vi "NaI_Readout_tdms.vi"() -> ()   [LabVIEW 2016]
doc: "Example: Configured Acquisition Auto TRIG\n\nRecommended Input Signal: 100 kHz, 4 Vpp, sine wave\n\nDevices Supported: NI 5102, NI 5911, NI 5112, NI 5620 \n(NI 5620 requires configuring 50 ohm input impedance and a 2 V vertical range)\n\nDescription:\n\nThis example is the same as the configured acquisition example included with the shipping examples, except this VI will use an immediate trigger if a timeout error is returned because no trigger is present. If a timeout occurs the code aborts and resets the session, while setting the trigger source to immediate. This example allows you use any of the available trigger sources, rather than just edge trigger as in the AutoSetup VI."
uses:
  <instrlib>/niScope/Acquire/Fetch/niScope Multi Fetch.vi
panel:
  out "Histogram":dynamicdata(graph)
  in  "resource name":refnum<k15>="PXI1Slot8"
  in  "Operator":string="Hsin-Yeh"
  in  "Target Total Events":i32=10000
  in  "file path":path=path "C:/Users/NTU/Desktop/Chih-Ping/NaI0827/1-haveNumber/Co60/Co60_5.tdms"
  out "Waveform from Digitizer vs. Sample Number":dbl[][](graph)=[[-0.007034295140918245, -0.005815471424873819, -0.004596647708829393, -0.0033778239927849674, -0.0033778239927849674, -0.004596647708829393, -0.007034295140918245, -0.0033778239927849674, -0.005815471424873819, -0.0033778239927849674, -0.0021590002767405414, -0.005815471424873819, -0.005815471424873819, -0.004596647708829393, -0.005815471424873819, -0.004596647708829393, -0.007034295140918245, -0.0021590002767405414, -0.005815471424873819, -0.005815471424873819, -0.0033778239927849674, -0.004596647708829393, -0.004596647708829393, -0.004596647708829393, -0.0033778239927849674, -0.0021590002767405414, -0.007034295140918245, -0.004596647708829393, -0.0033778239927849674, -0.004596647708829393, -0.0021590002767405414, -0.007034295140918245, -0.004596647708829393, -0.005815471424873819, -0.0033778239927849674, -0.0033778239927849674, -0.004596647708829393, -0.004596647708829393, -0.005815471424873819, -0.004596647708829393, -0.008253118856962671, -0.004596647708829393, -0.004596647708829393, -0.004596647708829393, -0.004596647708829393, -0.007034295140918245, -0.007034295140918245, -0.005815471424873819, -0.007034295140918245, -0.004596647708829393, -0.005815471424873819, -0.004596647708829393, -0.004596647708829393, -0.0021590002767405414, -0.007034295140918245, 0.0002786471553483105, -0.005815471424873819, -0.005815471424873819, -0.0033778239927849674, -0.005815471424873819, -0.004596647708829393, -0.004596647708829393, -0.005815471424873819, -0.005815471424873819, -0.005815471424873819, -0.005815471424873819, -0.0033778239927849674, -0.007034295140918245, -0.004596647708829393, -0.004596647708829393, -0.004596647708829393, -0.0033778239927849674, -0.005815471424873819, -0.0033778239927849674, -0.004596647708829393, -0.005815471424873819, -0.005815471424873819, -0.0021590002767405414, -0.004596647708829393, -0.004596647708829393, -0.004596647708829393, -0.0033778239927849674, -0.009471942573007097, -0.004596647708829393, -0.007034295140918245, -0.004596647708829393, -0.007034295140918245, -0.0033778239927849674, -0.0033778239927849674, -0.004596647708829393, -0.005815471424873819, -0.0021590002767405414, -0.005815471424873819, -0.005815471424873819, -0.004596647708829393, -0.004596647708829393, -0.007034295140918245, -0.0033778239927849674, -0.005815471424873819, -0.008253118856962671, -0.007034295140918245, -0.004596647708829393, -0.0033778239927849674, -0.004596647708829393, -0.008253118856962671, -0.0033778239927849674, -0.007034295140918245, -0.0033778239927849674, -0.0033778239927849674, -0.004596647708829393, -0.007034295140918245, -0.004596647708829393, -0.0033778239927849674, -0.007034295140918245, -0.004596647708829393, -0.004596647708829393, -0.007034295140918245, -0.004596647708829393, -0.005815471424873819, -0.004596647708829393, -0.007034295140918245, -0.004596647708829393, -0.004596647708829393, -0.0033778239927849674, -0.005815471424873819, -0.007034295140918245, -0.005815471424873819, -0.005815471424873819, -0.004596647708829393, -0.005815471424873819, -0.004596647708829393, -0.0033778239927849674, -0.0033778239927849674, -0.005815471424873819, -0.005815471424873819, -0.004596647708829393, -0.004596647708829393, -0.005815471424873819, -0.004596647708829393, -0.005815471424873819, -0.005815471424873819, -0.0021590002767405414, -0.0033778239927849674, -0.004596647708829393, -0.007034295140918245, -0.005815471424873819, -0.005815471424873819, -0.004596647708829393, -0.007034295140918245, -0.005815471424873819, -0.0033778239927849674, -0.0009401765606961154, -0.004596647708829393, -0.004596647708829393, -0.0033778239927849674, -0.0021590002767405414, -0.005815471424873819, -0.004596647708829393, -0.005815471424873819, 0.008810413167659292, 0.06000100924152518, 0.07584571755010272, 0.08559630727845813, 0.08803395471054698, 0.09169042585868026, 0.08803395471054698, 0.0892527784265914, 0.08803395471054698, 0.09169042585868026, 0.09290924957472468, 0.0892527784265914, 0.08803395471054698, 0.09047160214263583, 0.0892527784265914, 0.09169042585868026, 0.08681513099450255, 0.0892527784265914, 0.08803395471054698, 0.08559630727845813, 0.08681513099450255, 0.0892527784265914, 0.08803395471054698, 0.08315865984636928, 0.08559630727845813, 0.08559630727845813, 0.08559630727845813, 0.08315865984636928, 0.08559630727845813, 0.0843774835624137, 0.08315865984636928, 0.08193983613032485, 0.08315865984636928, 0.0843774835624137, 0.079502188698236, 0.08315865984636928, 0.079502188698236, 0.0843774835624137, 0.0843774835624137, 0.079502188698236, 0.07828336498219157, 0.08072101241428042, 0.079502188698236, 0.07828336498219157, 0.079502188698236, 0.07706454126614715, 0.07706454126614715, 0.079502188698236, 0.079502188698236, 0.07828336498219157, 0.0746268938340583, 0.07828336498219157, 0.07584571755010272, 0.07218924640196944, 0.079502188698236, 0.07340807011801387, 0.07584571755010272, 0.0746268938340583, 0.07340807011801387, 0.07218924640196944, 0.07340807011801387, 0.07218924640196944, 0.07340807011801387, 0.07097042268592502, 0.07097042268592502, 0.0746268938340583, 0.07218924640196944, 0.07097042268592502, 0.07340807011801387, 0.06975159896988059, 0.06853277525383616, 0.07340807011801387, 0.06731395153779174, 0.07097042268592502, 0.06975159896988059, 0.07097042268592502, 0.06853277525383616, 0.06853277525383616, 0.06731395153779174, 0.06731395153779174, 0.06609512782174731, 0.06609512782174731, 0.06609512782174731, 0.06975159896988059, 0.06487630410570289, 0.06487630410570289, 0.06731395153779174, 0.06609512782174731, 0.06487630410570289, 0.062438656673614035, 0.06365748038965846, 0.06731395153779174, 0.06731395153779174, 0.062438656673614035, 0.06000100924152518, 0.06121983295756961, 0.06121983295756961, 0.06365748038965846, 0.06365748038965846, 0.062438656673614035, 0.06000100924152518, 0.062438656673614035, 0.06121983295756961, 0.05878218552548076, 0.05878218552548076, 0.06121983295756961, 0.05878218552548076, 0.06121983295756961, 0.06000100924152518, 0.06000100924152518, 0.05756336180943633, 0.05878218552548076, 0.05878218552548076, 0.056344538093391905, 0.056344538093391905, 0.05756336180943633, 0.06000100924152518, 0.05756336180943633, 0.05878218552548076, 0.06000100924152518, 0.056344538093391905, 0.056344538093391905, 0.05512571437734748, 0.05512571437734748, 0.05512571437734748, 0.05512571437734748, 0.05512571437734748, 0.05268806694525863, 0.05390689066130305, 0.05268806694525863, 0.05512571437734748, 0.0514692432292142, 0.05390689066130305, 0.0514692432292142, 0.05268806694525863, 0.05268806694525863, 0.05268806694525863, 0.0514692432292142, 0.050250419513169775, 0.04903159579712535, 0.04903159579712535, 0.04903159579712535, 0.050250419513169775, 0.05268806694525863, 0.050250419513169775, 0.050250419513169775, 0.050250419513169775, 0.0514692432292142, 0.044156300932947645, 0.0514692432292142, 0.0465939483650365, 0.0514692432292142, 0.0465939483650365, 0.04903159579712535, 0.050250419513169775, 0.044156300932947645, 0.04903159579712535, 0.04781277208108092, 0.04781277208108092, 0.04903159579712535, 0.0465939483650365, 0.04171865350085879, 0.0465939483650365, 0.04537512464899207, 0.0465939483650365, 0.044156300932947645, 0.04781277208108092, 0.04537512464899207, 0.044156300932947645, 0.044156300932947645, 0.04781277208108092, 0.04171865350085879, 0.04171865350085879, 0.04293747721690322, 0.04293747721690322, 0.04171865350085879, 0.044156300932947645, 0.04293747721690322, 0.04171865350085879, 0.038062182352725515, 0.04537512464899207, 0.04293747721690322, 0.04049982978481437, 0.04293747721690322, 0.03928100606876994, 0.04293747721690322, 0.04049982978481437, 0.04171865350085879, 0.03928100606876994, 0.04049982978481437, 0.04049982978481437, 0.04049982978481437, 0.04171865350085879, 0.04049982978481437, 0.03928100606876994, 0.03928100606876994, 0.03928100606876994, 0.04171865350085879, 0.04049982978481437, 0.038062182352725515, 0.03684335863668109, 0.03684335863668109, 0.03928100606876994, 0.038062182352725515, 0.035624534920636663, 0.038062182352725515, 0.03928100606876994, 0.038062182352725515, 0.03684335863668109, 0.03318688748854781, 0.03928100606876994, 0.03684335863668109, 0.03318688748854781, 0.035624534920636663, 0.035624534920636663, 0.03684335863668109, 0.03440571120459224, 0.03684335863668109, 0.035624534920636663, 0.03440571120459224, 0.03440571120459224, 0.03684335863668109, 0.03318688748854781, 0.035624534920636663, 0.03318688748854781, 0.038062182352725515, 0.035624534920636663, 0.035624534920636663, 0.03440571120459224, 0.03318688748854781, 0.03440571120459224, 0.03440571120459224, 0.03318688748854781, 0.03318688748854781, 0.03318688748854781, 0.03318688748854781, 0.03318688748854781, 0.03074924005645896, 0.03074924005645896, 0.029530416340414534, 0.029530416340414534, 0.03318688748854781, 0.031968063772503386, 0.028311592624370108, 0.031968063772503386, 0.029530416340414534, 0.03074924005645896, 0.027092768908325682, 0.03074924005645896, 0.03074924005645896, 0.031968063772503386, 0.031968063772503386, 0.027092768908325682, 0.029530416340414534, 0.03074924005645896, 0.02465512147623683, 0.028311592624370108, 0.029530416340414534, 0.029530416340414534, 0.029530416340414534, 0.03074924005645896, 0.027092768908325682, 0.028311592624370108, 0.027092768908325682, 0.029530416340414534, 0.027092768908325682, 0.02465512147623683, 0.031968063772503386, 0.027092768908325682, 0.027092768908325682, 0.027092768908325682, 0.02465512147623683, 0.028311592624370108, 0.02465512147623683, 0.025873945192281256, 0.025873945192281256, 0.023436297760192404, 0.027092768908325682, 0.023436297760192404, 0.025873945192281256, 0.025873945192281256, 0.02465512147623683, 0.028311592624370108, 0.027092768908325682, 0.027092768908325682, 0.023436297760192404, 0.022217474044147978, 0.025873945192281256, 0.02465512147623683, 0.023436297760192404, 0.027092768908325682, 0.023436297760192404, 0.023436297760192404, 0.022217474044147978, 0.027092768908325682, 0.02465512147623683, 0.02465512147623683, 0.02465512147623683, 0.023436297760192404, 0.02465512147623683, 0.02465512147623683, 0.02465512147623683, 0.022217474044147978, 0.02465512147623683, 0.02465512147623683, 0.02465512147623683, 0.02465512147623683, 0.022217474044147978, 0.022217474044147978, 0.020998650328103552, 0.017342179179970274, 0.020998650328103552, 0.019779826612059126, 0.020998650328103552, 0.0185610028960147, 0.022217474044147978, 0.020998650328103552, 0.023436297760192404, 0.019779826612059126, 0.019779826612059126, 0.022217474044147978, 0.017342179179970274, 0.0185610028960147, 0.0185610028960147, 0.019779826612059126, 0.014904531747881422, 0.019779826612059126, 0.02465512147623683, 0.019779826612059126, 0.019779826612059126, 0.020998650328103552, 0.019779826612059126, 0.016123355463925848, 0.019779826612059126, 0.020998650328103552, 0.017342179179970274, 0.0185610028960147, 0.0185610028960147, 0.017342179179970274, 0.0185610028960147, 0.020998650328103552, 0.0185610028960147, 0.019779826612059126, 0.017342179179970274, 0.014904531747881422, 0.016123355463925848, 0.017342179179970274, 0.0185610028960147, 0.016123355463925848, 0.017342179179970274, 0.017342179179970274, 0.017342179179970274, 0.0185610028960147, 0.019779826612059126, 0.014904531747881422, 0.019779826612059126, 0.013685708031836996, 0.016123355463925848, 0.017342179179970274, 0.014904531747881422, 0.017342179179970274, 0.016123355463925848, 0.017342179179970274, 0.014904531747881422, 0.014904531747881422, 0.013685708031836996, 0.017342179179970274, 0.016123355463925848, 0.013685708031836996, 0.017342179179970274, 0.0185610028960147, 0.014904531747881422, 0.016123355463925848, 0.013685708031836996, 0.017342179179970274, 0.01246688431579257, 0.014904531747881422, 0.014904531747881422, 0.014904531747881422, 0.014904531747881422, 0.014904531747881422, 0.013685708031836996, 0.013685708031836996, 0.016123355463925848, 0.01246688431579257, 0.013685708031836996, 0.013685708031836996, 0.013685708031836996, 0.013685708031836996, 0.014904531747881422, 0.014904531747881422, 0.01246688431579257, 0.01246688431579257, 0.013685708031836996, 0.014904531747881422, 0.013685708031836996, 0.013685708031836996, 0.013685708031836996, 0.01246688431579257, 0.017342179179970274, 0.016123355463925848, 0.013685708031836996, 0.016123355463925848, 0.01246688431579257, 0.013685708031836996, 0.014904531747881422, 0.01246688431579257, 0.010029236883703718, 0.013685708031836996, 0.010029236883703718, 0.010029236883703718, 0.014904531747881422, 0.013685708031836996, 0.014904531747881422, 0.011248060599748144, 0.008810413167659292, 0.011248060599748144, 0.01246688431579257, 0.013685708031836996, 0.008810413167659292, 0.013685708031836996, 0.01246688431579257, 0.01246688431579257, 0.01246688431579257, 0.01246688431579257, 0.008810413167659292, 0.013685708031836996, 0.013685708031836996, 0.010029236883703718, 0.008810413167659292, 0.011248060599748144, 0.01246688431579257, 0.01246688431579257, 0.008810413167659292, 0.01246688431579257, 0.010029236883703718, 0.013685708031836996, 0.00637276573557044, 0.007591589451614866, 0.010029236883703718, 0.010029236883703718, 0.010029236883703718, 0.008810413167659292, 0.01246688431579257, 0.011248060599748144, 0.010029236883703718, 0.008810413167659292, 0.008810413167659292, 0.011248060599748144, 0.007591589451614866, 0.010029236883703718, 0.008810413167659292, 0.00637276573557044, 0.008810413167659292, 0.01246688431579257, 0.008810413167659292, 0.01246688431579257, 0.011248060599748144, 0.008810413167659292, 0.008810413167659292, 0.007591589451614866, 0.008810413167659292, 0.00637276573557044, 0.010029236883703718, 0.010029236883703718, 0.005153942019526014, 0.00637276573557044, 0.007591589451614866, 0.007591589451614866, 0.008810413167659292, 0.008810413167659292, 0.010029236883703718, 0.008810413167659292, 0.008810413167659292, 0.007591589451614866, 0.007591589451614866, 0.007591589451614866, 0.00637276573557044, 0.00637276573557044, 0.010029236883703718, 0.00637276573557044, 0.007591589451614866, 0.007591589451614866, 0.010029236883703718, 0.010029236883703718, 0.011248060599748144, 0.008810413167659292, 0.005153942019526014, 0.007591589451614866, 0.00637276573557044, 0.00637276573557044, 0.00637276573557044, 0.005153942019526014, 0.007591589451614866, 0.007591589451614866, 0.007591589451614866, 0.007591589451614866, 0.01246688431579257, 0.00637276573557044, 0.007591589451614866, 0.008810413167659292, 0.005153942019526014, 0.005153942019526014, 0.008810413167659292, 0.00637276573557044, 0.00637276573557044, 0.00637276573557044, 0.005153942019526014, 0.003935118303481588, 0.005153942019526014, 0.007591589451614866, 0.0014974708713927365, 0.005153942019526014, 0.005153942019526014, 0.005153942019526014, 0.007591589451614866, 0.003935118303481588, 0.005153942019526014, 0.003935118303481588, 0.008810413167659292, 0.003935118303481588, 0.003935118303481588, 0.003935118303481588, 0.00637276573557044, 0.005153942019526014, 0.005153942019526014, 0.005153942019526014, 0.005153942019526014, 0.007591589451614866, 0.00637276573557044, 0.00637276573557044, 0.005153942019526014, 0.00637276573557044, 0.00637276573557044, 0.00637276573557044, 0.003935118303481588, 0.003935118303481588, 0.005153942019526014, 0.005153942019526014, 0.005153942019526014, 0.008810413167659292, 0.0027162945874371625, 0.005153942019526014, 0.005153942019526014, 0.0027162945874371625, 0.003935118303481588, 0.005153942019526014, 0.003935118303481588, 0.0014974708713927365, 0.003935118303481588, 0.00637276573557044, 0.005153942019526014, 0.00637276573557044, 0.0027162945874371625, 0.003935118303481588, 0.0027162945874371625, 0.003935118303481588, 0.003935118303481588, 0.0027162945874371625, 0.007591589451614866, 0.005153942019526014, 0.003935118303481588, 0.003935118303481588, 0.005153942019526014, 0.003935118303481588, 0.0027162945874371625, 0.005153942019526014, 0.0027162945874371625, 0.00637276573557044, -0.0009401765606961154, 0.003935118303481588, 0.005153942019526014, 0.005153942019526014, 0.003935118303481588, 0.005153942019526014, 0.0002786471553483105, 0.0002786471553483105, 0.003935118303481588, 0.0014974708713927365, 0.0027162945874371625, 0.0027162945874371625, 0.0014974708713927365, 0.0027162945874371625, 0.0027162945874371625, 0.0014974708713927365, 0.0014974708713927365, 0.003935118303481588, 0.0027162945874371625, 0.0014974708713927365, 0.0027162945874371625, 0.0027162945874371625, 0.0027162945874371625, 0.005153942019526014, 0.0027162945874371625, 0.0014974708713927365, 0.003935118303481588, -0.0021590002767405414, 0.0002786471553483105, 0.005153942019526014, 0.0002786471553483105, 0.0027162945874371625, 0.0027162945874371625, 0.003935118303481588, 0.0027162945874371625, 0.0014974708713927365, -0.0009401765606961154, 0.0002786471553483105, 0.003935118303481588, 0.0002786471553483105, 0.0014974708713927365, 0.005153942019526014, 0.0027162945874371625, 0.0027162945874371625, 0.0027162945874371625, 0.003935118303481588, 0.003935118303481588, 0.0002786471553483105, 0.0027162945874371625, 0.0002786471553483105, 0.0014974708713927365, -0.0021590002767405414, 0.003935118303481588, 0.0027162945874371625, 0.0014974708713927365, 0.0027162945874371625, 0.0002786471553483105, 0.0014974708713927365, 0.0014974708713927365, 0.0002786471553483105, 0.0014974708713927365, 0.0014974708713927365, -0.0009401765606961154, 0.0014974708713927365, 0.0002786471553483105, 0.0014974708713927365, 0.0002786471553483105, 0.0002786471553483105, 0.0014974708713927365, 0.0014974708713927365, 0.0002786471553483105, -0.0009401765606961154]]
  out "Event rate (Hz)":dbl=73.3159330185636
  in  "reference position":dbl=20.0 caption="Ref Position" format="%.1f"
  out "Event Number":dbl=10000.0
  in  "Don't Write Data":bool
  in  "trigger coupling":i32(slide)=1 caption="Trigger Coupling"
  in  "trigger level":dbl=0.03 caption="Trigger Level" format="%.2f"
  in  "trigger holdoff":dbl caption="Trigger Holdoff" format="%^.4e"
  in  "trigger delay":dbl caption="Trigger Delay" format="%^.4e"
  in  "trigger slope":i32(ring) caption="Trigger Slope" items=["Positive", "Negative"]
  in  "trigger source":string(combo)="0" caption="Trigger Source"
  in  "maximum input frequency":dbl=1000000000.0 caption="Max. Input Frequency" format="%.2f"
  in  "input impedance":u32(ring)=2 caption="Input Impedance" items=["1 mega ohm", "75 ohms", "50 ohms"]
  in  "vertical coupling":u32(slide)=1 caption="Vertical\nCcoupling"
  in  "probe attenuation":dbl=1.0 caption="Probe Attenuation" format="%.1f"
  in  "vertical offset":dbl=0.5 caption="Vertical Offset" format="%.4f"
  in  "trigger type":enum16{"Edge"}(ring) caption="Trigger Type"
  out "actual sample rate":dbl=5000000.0 caption="Actual Sample Rate" format="%^.2e"
  out "actual record length":i32=800 caption="Actual Record Length"
  in  "?":bool
  in  "min record length":i32=800 caption="Min. Record Length"
  in  "min sample rate":dbl=5000000.0 caption="Min. Sample Rate" step=1000000.0 format="%^.2e"
  in  "vertical range":dbl=1.0 caption="Vertical Range (V)" format="%.2f"
  in  "channel name":string="0" caption="Channel Name(s)"
  # "Vertical"
  # "Channel"
  # "Trigger"
  # "Trigger Selection"
  # "Specific Parameters - Not all parameters \napply to all trigger types."
  # "Horizontal"
  # "Common Parameters"
  # "NI PXIe 5162 Spec : 1.5 GHz, 5 GS/s, 10-Bit\nhttps://www.ni.com/pdf/manuals/373858j.pdf"
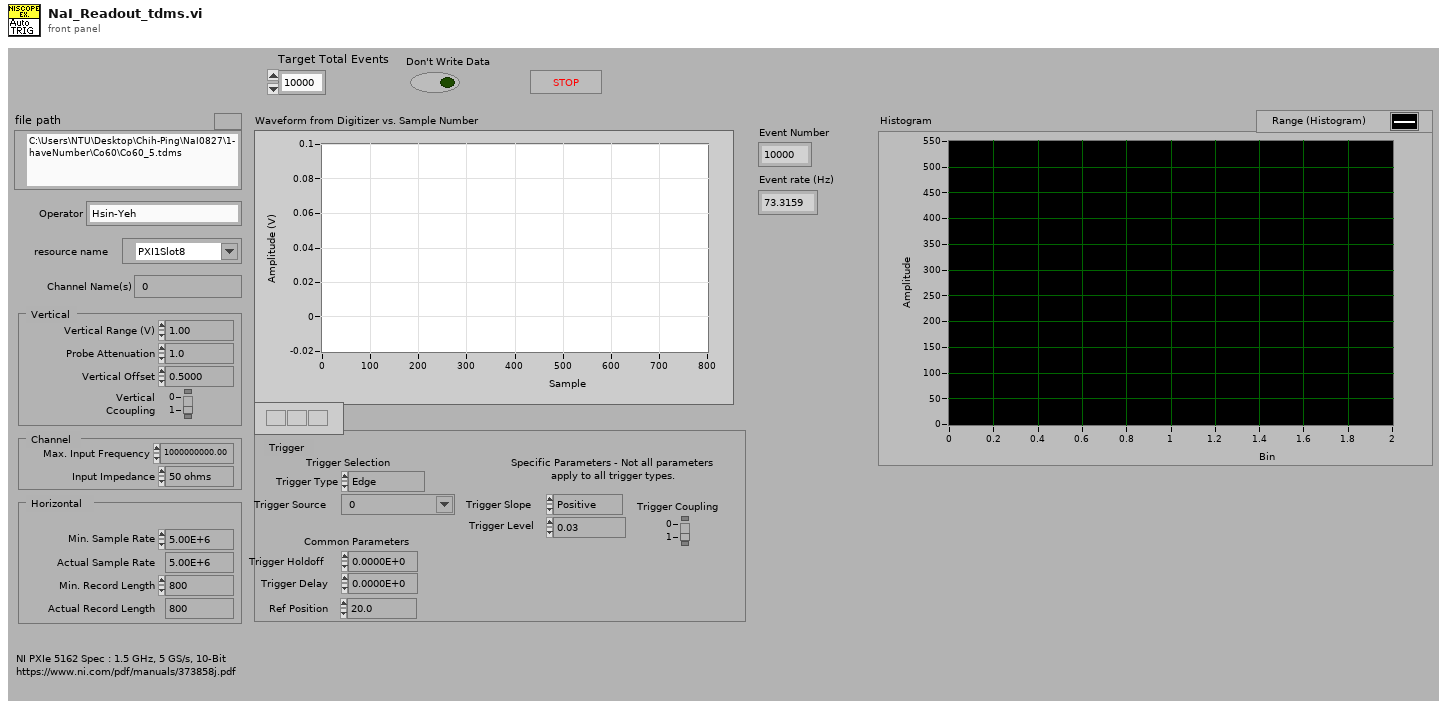
[diagram p1: front panel]
types:
  T1 = enum16{"open", "open or create", "create or replace", "create", "open (read-only)"}
  T2 = enum16{"Edge", "Hysteresis", "Digital", "Window", "Immediate"}
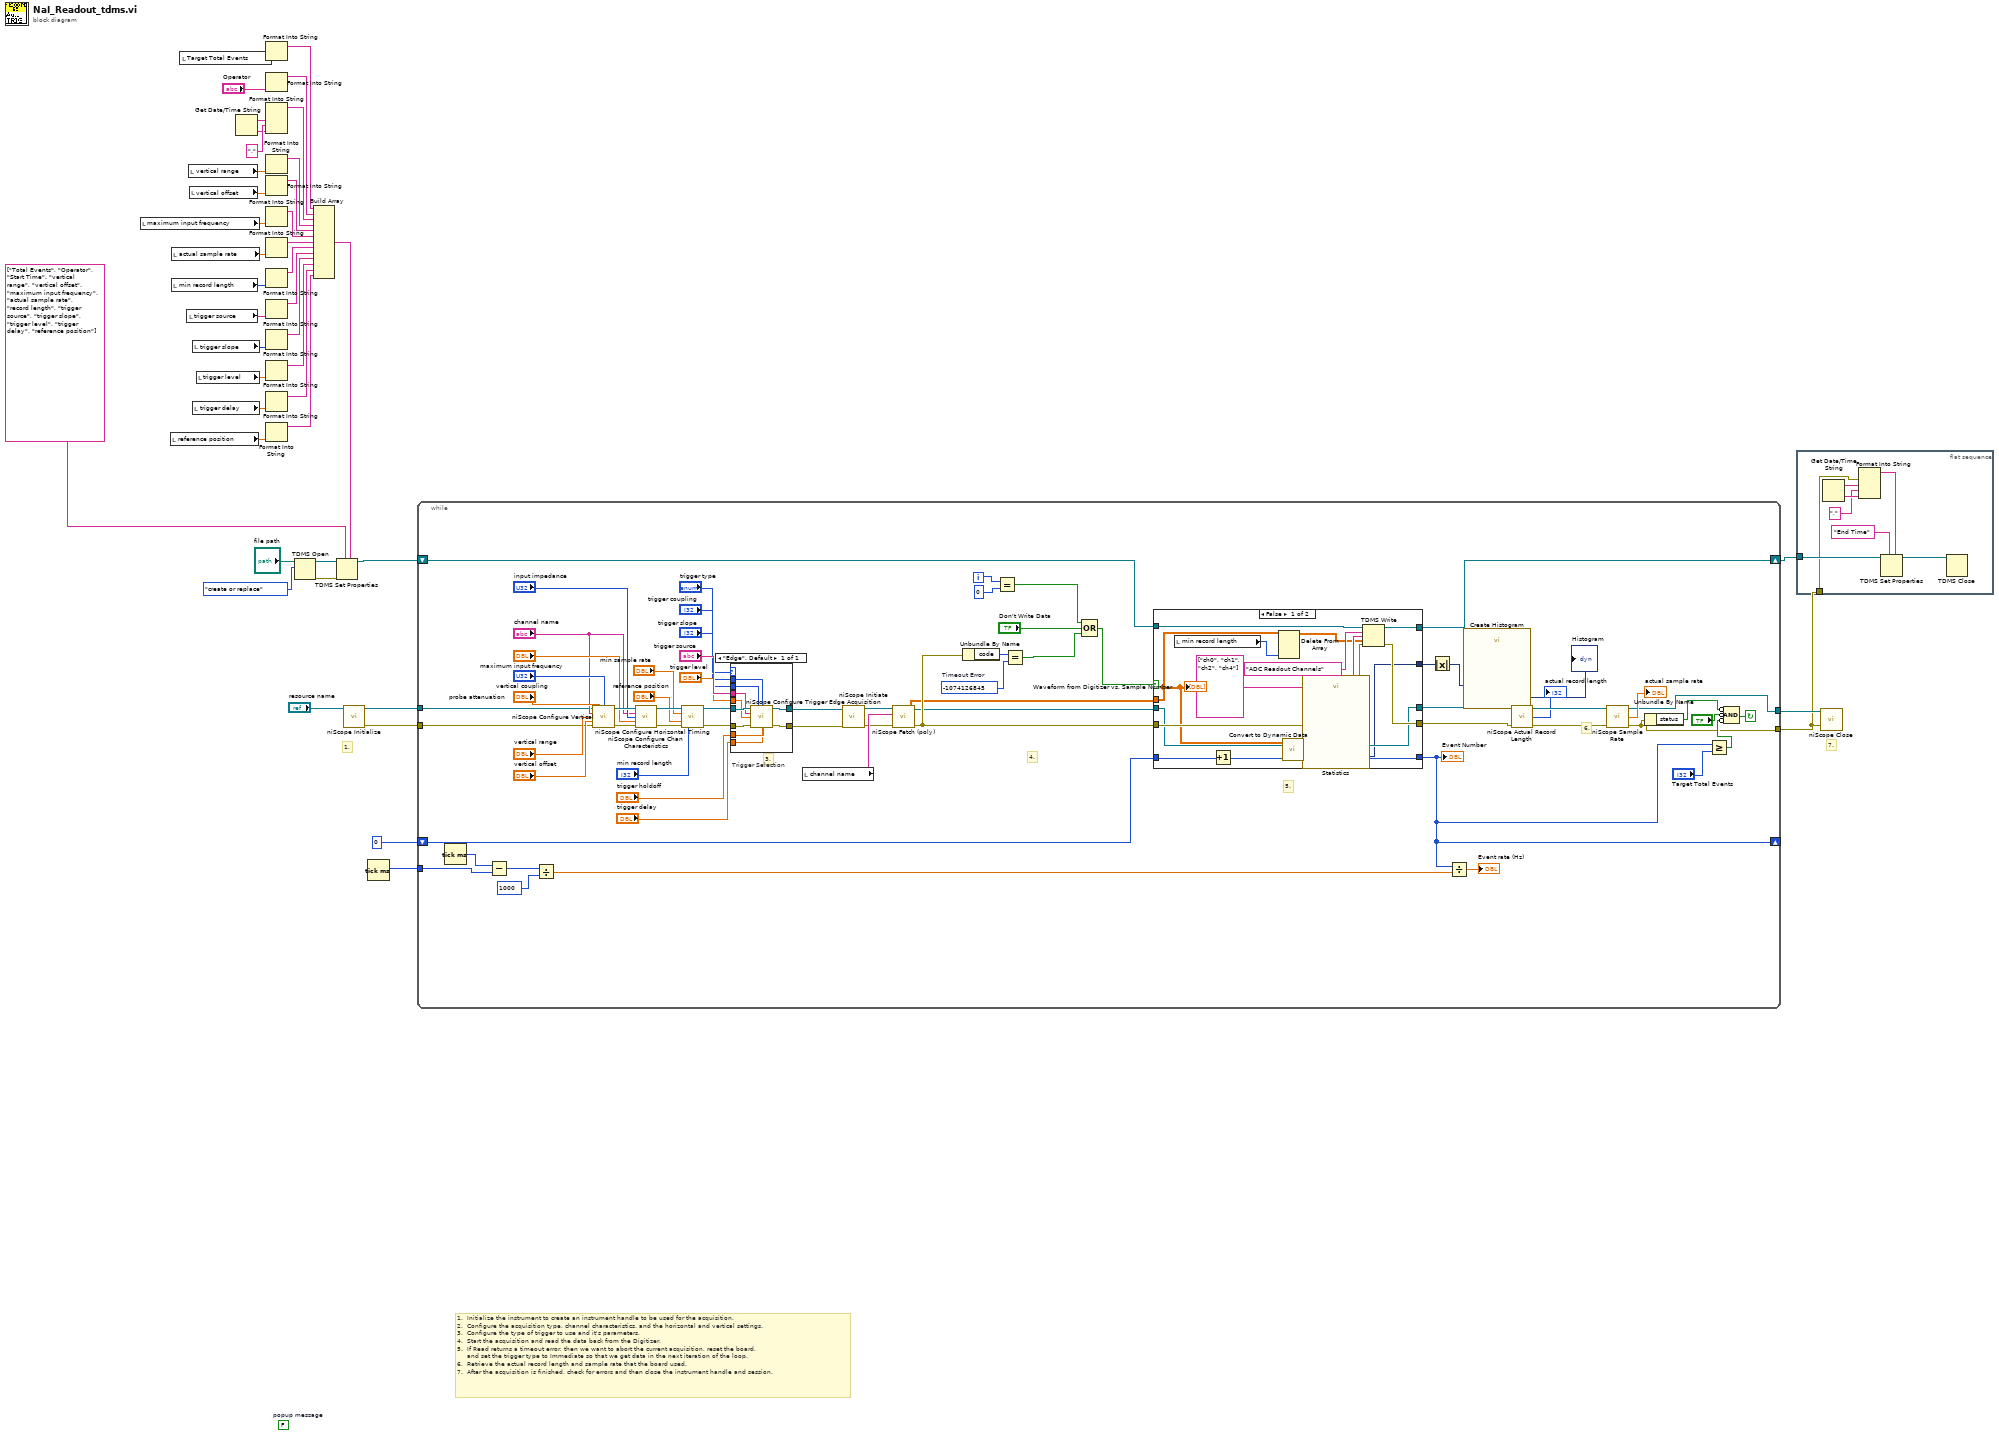
[diagram p0: block diagram]
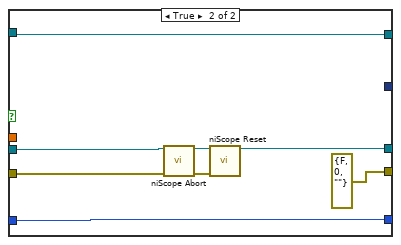
[diagram p2: hidden frame]
diagram:
  (unwired) FALSE  # popup message
  # "1.  Initialize the instrument to create an instrument handle to be used for the acquisition.\n2.  Configure the acquisition type, channel characteristics, and the horizontal and vertical settings.\n3.  Configure the type of trigger to use and it's parameters.\n4.  Start the acquisition and read the data back from the Digitizer.\n5.  If Read returns a timeout error, then we want to abort the current acquisition, reset the board,\n     and set the trigger type to Immediate so that we get data in the next iteration of the loop.\n6.  Retrieve the actual record length and sample rate that the board used.\n7.  After the acquisition is finished, check for errors and then close the instrument handle and session."
  # "7."
  # "1."
  n1 = local read "maximum input frequency"() -> (w25:dbl)
  n2 = local read "reference position"() -> (w27:dbl)
  n3 = local read "actual sample rate"() -> (w29:dbl)
  n4 = local read "min record length"() -> (w32:i32)
  n5 = local read "Target Total Events"() -> (w35:i32)
  n6 = local read "trigger source"() -> (w31:string)
  n7 = local read "vertical range"() -> (w30:dbl)
  n8 = local read "vertical offset"() -> (w26:dbl)
  n9 = local read "trigger slope"() -> (w17:i32)
  n10 = local read "trigger delay"() -> (w28:dbl)
  n11 = local read "trigger level"() -> (w33:dbl)
  n12 = Get Date/Time String() -> (date string=w23:string, time string=w21:string)  [unwired: 3 in]
  n13 = Format Into String(w35) -> (resulting string=w34:string)  [unwired: 3 in, 1 out]
  n14 = Format Into String("Operator") -> (resulting string=w20:string)  [unwired: 3 in, 1 out]
  n15 = Format Into String(w23, "," ("input 2"), w21) -> (resulting string=w19:string)  [unwired: 3 in, 1 out]
  n16 = Format Into String(w30) -> (resulting string=w18:string)  [unwired: 3 in, 1 out]
  n17 = Format Into String(w26) -> (resulting string=w15:string)  [unwired: 3 in, 1 out]
  n18 = Format Into String(w25) -> (resulting string=w16:string)  [unwired: 3 in, 1 out]
  n19 = Format Into String(w29) -> (resulting string=w14:string)  [unwired: 3 in, 1 out]
  n20 = Format Into String(w32) -> (resulting string=w13:string)  [unwired: 3 in, 1 out]
  n21 = Format Into String(w31) -> (resulting string=w12:string)  [unwired: 3 in, 1 out]
  n22 = Format Into String(w17) -> (resulting string=w11:string)  [unwired: 3 in, 1 out]
  n23 = Format Into String(w33) -> (resulting string=w10:string)  [unwired: 3 in, 1 out]
  n24 = Format Into String(w28) -> (resulting string=w9:string)  [unwired: 3 in, 1 out]
  n25 = Format Into String(w27) -> (resulting string=w8:string)  [unwired: 3 in, 1 out]
  n26 = TDMS Open(10:T1."create or replace" ("operation (0:open)"), 11:"file path") -> (0:w37:errorcluster, 3:w36:refnum<k34>)  [unwired: 5 in]
  n27 = Build Array(w34, w20, w19, w18, w15, w16, w14, w13, w12, w11, w10, w9, w8) -> (w7:string[])
  n28 = TDMS Set Properties(5:w7, 7:string[] ["Total Events", "Operator", "Start Time", "vertical range", "vertical offset", "maximum input frequency", "actual sample rate", "record length", "trigger source", "trigger slope", "trigger level", "trigger delay", "reference position"] ("property names"), 8:w37, 11:w36) -> (3:w5:refnum<k34>)  [unwired: 2 in, 3 out]
  n29 = call <instrlib>:"niScope Initialize.vi"("resource name"="resource name") -> ("instrument handle"=w43:refnum<k15>, "error out"=w42:errorcluster)  [unwired: 13 in]
  n30 = Tick Count (ms)() -> (millisecond timer value=w40:u32)
  n31 = while {
    tunnel: w42 -> [w75]
    tunnel: w43 -> [w76]
    shift-right: [w50] -> _
    shift-left: 0 -> [w66]
    tunnel: w40 -> [w71]
    shift-right: [w63] -> w4
    shift-left: w5 -> [w64]
    tunnel: [w49] -> w3
    tunnel: [w48] -> w2
    i -> [w61]
    stop <- w85 continue-if-true
    w83 = -1074126845  # Timeout Error
    # "6."
    # "5."
    # "4."
    # "3."
    # "2."
    # "Data Acquisition Loop"
    n32 = Tick Count (ms)() -> (millisecond timer value=w70:u32)
    n33 = Subtract(x=w70, y=w71) -> (x-y=w69:u32)
    n34 = Divide(x=w69, y=u32 1000) -> (x/y=w67:dbl)
    n35 = call <instrlib>:"niScope Configure Vertical.vi"("instrument handle"=w76, "probe attenuation"="probe attenuation", "vertical coupling"="vertical coupling", "channels"="channel name", "vertical range"="vertical range", "vertical offset"="vertical offset", "error in"=w75) -> ("instrument handle out"=w104:refnum<k15>, "error out"=w103:errorcluster)  [unwired: 7 in]
    n36 = call <instrlib>:"niScope Configure Chan Characteristics.vi"("instrument handle"=w104, "channels"="channel name", "input impedance"="input impedance", "maximum input frequency"="maximum input frequency", "error in"=w103) -> ("instrument handle out"=w101:refnum<k15>, "error out"=w102:errorcluster)  [unwired: 9 in]
    n37 = call <instrlib>:"niScope Configure Horizontal Timing.vi"("instrument handle"=w101, "min sample rate"="min sample rate", "reference position"="reference position", "error in"=w102, "min record length"="min record length") -> ("instrument handle out"=w94:refnum<k15>, "error out"=w95:errorcluster)  [unwired: 9 in]
    n38 = case "Trigger Selection" shown="\"Edge\", Default" "trigger type" {
      tunnel: w95 -> [w143]
      tunnel: [w137] -> w53
      tunnel: w94 -> [w142]
      tunnel: [w138] -> w78
      tunnel: "trigger source" -> [w141]
      tunnel: "trigger holdoff" -> [w140]
      tunnel: "trigger delay" -> [w139]
      tunnel: "trigger level" -> [w136]
      tunnel: "trigger slope" -> [w135]
      tunnel: "trigger coupling" -> [w134]
      frame "Edge", Default {
        n39 = call <instrlib>:"niScope Configure Trigger Edge.vi"("instrument handle"=w142, "trigger slope"=w135, "trigger coupling"=w134, "trigger source"=w141, "trigger level"=w136, "error in"=w143, "trigger holdoff"=w140, "trigger delay"=w139) -> ("instrument handle out"=w138:refnum<k15>, "error out"=w137:errorcluster)  [unwired: 6 in]
      }
    }
    n40 = local read "channel name"() -> (w54:string)
    n41 = call <instrlib>:"niScope Initiate Acquisition.vi"("instrument handle"=w78, "error in"=w53) -> ("instrument handle out"=w77:refnum<k15>, "error out"=w52:errorcluster)  [unwired: 12 in]
    n42 = call-poly <instrlib>:"niScope Fetch (poly).vi"("error in"=w52, "channels"=w54, "instrument handle"=w77) -> ("error out"=w80:errorcluster, "wfm"=w72:dbl[][], "instrument handle out"=w79:refnum<k15>)  [unwired: 5 in, 1 out]
    n43 = Unbundle By Name(w80) -> ("code"=w82:i32)
    n44 = Equal?(x=w61, y=0) -> (x = y?=w59:bool)
    n45 = Equal?(x=w82, y=w83) -> (x = y?=w57:bool)
    n46 = Compound Arithmetic op=OR(w59, "Don't Write Data", w57) -> (w56:bool)
    n47 = case shown="False" w56 {
      tunnel: w80 -> [w121 w133]
      tunnel: w79 -> [w114 w132]
      tunnel: [w114 w129] -> w51
      tunnel: [w119 errorcluster {"status"=FALSE, "code"=0, "source"=""} ("error out")] -> w47
      tunnel: w72 -> [w113 _]
      tunnel: [w120 w126] -> w63
      tunnel: w66 -> [w124 w125]
      tunnel: [w123 w125] -> w50
      tunnel: w64 -> [w122 w126]
      tunnel: [w111 _] -> w44
      frame False {
        n48 = local read "min record length"() -> (w115:i32)
        n49 = Increment(x=w124) -> (x+1=w123:i32)
        n50 = Delete From Array(array=w113, index (col)=w115) -> (array with subset deleted=w116:dbl[][])  [unwired: 2 in, 1 out]
        n51 = call "Convert to Dynamic Data"("2D Array"=w113) -> ("Dynamic Data Type"=w112:dynamicdata)  [unwired: 3 in]
        n52 = call "Statistics"("Signals"=w112) -> ("Range"=w111:dynamicdata)  [unwired: 23 in, 3 out]
        n53 = TDMS Write(0:w122, 5:"ADC Readout Channels" ("group name (Untitled)"), 7:string[] ["ch0", "ch1", "ch2", "ch4"] ("channel name(s)"), 9:w116, 11:w121) -> (4:w120:refnum<k34>, 15:w119:errorcluster)  [unwired: 1 in, 2 out]
        "Waveform from Digitizer vs. Sample Number" <- w113
      }
      frame True {
        n54 = local write "trigger type"(T2."Edge" ("trigger type")) -> ()
        n55 = call <instrlib>:"niScope Abort.vi"("instrument handle"=w132, "error in"=w133) -> ("instrument handle out"=w131:refnum<k15>, "error out"=w130:errorcluster)  [unwired: 12 in]
        n56 = call <instrlib>:"niScope Reset.vi"("instrument handle"=w131, "error in"=w130) -> ("instrument handle out"=w129:refnum<k15>)  [unwired: 12 in, 1 out]
      }
    }
    "Event Number" <- w50
    n57 = Absolute Value(x=w44) -> (abs(x)=w45:dynamicdata)
    n58 = Divide(x=w50, y=w67) -> (x/y=→"Event rate (Hz)":dbl)
    n59 = call "Create Histogram"("Signal"=w45) -> ("Histogram"=→"Histogram":dynamicdata)  [unwired: 9 in, 1 out]
    n60 = call <instrlib>:"niScope Actual Record Length.vi"("instrument handle"=w51, "error in"=w47) -> ("instrument handle out"=w108:refnum<k15>, "actual record length"=→"actual record length":i32, "error out"=w107:errorcluster)  [unwired: 11 in]
    n61 = call <instrlib>:"niScope Sample Rate.vi"("instrument handle"=w108, "error in"=w107) -> ("instrument handle out"=w49:refnum<k15>, "actual sample rate"=→"actual sample rate":dbl, "error out"=w48:errorcluster)  [unwired: 11 in]
    n62 = Unbundle By Name(w48) -> ("status"=w84:bool)
    n63 = Greater Or Equal?(x=w50, y="Target Total Events") -> (x >= y?=w55:bool)
    n64 = Compound Arithmetic op=AND(invert w84, invert "?", invert w55) -> (w85:bool)
  }
  n65 = flat-sequence {
    tunnel: w4 -> [w151]
    tunnel: w2 -> [w144]
    frame #0 {
      n66 = Get Date/Time String() -> (date string=w149:string, time string=w148:string)  [unwired: 3 in]
      n67 = Format Into String(error in=w144, w149, "," ("input 2"), w148) -> (resulting string=w146:string)  [unwired: 2 in, 1 out]
      n68 = TDMS Set Properties(5:w146, 7:"End Time" ("input 2"), 11:w151) -> (3:w150:refnum<k34>)  [unwired: 3 in, 3 out]
      n69 = TDMS Close(11:w150) -> ()  [unwired: 1 in, 2 out]
    }
  }
  n70 = call <instrlib>:"niScope Close.vi"("instrument handle"=w3, "error in"=w2) -> ()  [unwired: 13 in, 1 out]
